vi "GUI.vi"() -> ()   [LabVIEW 2025]
uses:
  Data.ctl
  Case.ctl
  <vilib>/httpClient/ClientHandle.ctl
  User Connections/User Connections.lvclass
  Ini File/Ini File.lvclass
  D:/Repository/Semaphore-with-ESP32-C6/LabVIEW/User Connections/User Connections.lvclass
  <vilib>/JDP Science/JSONtext/Next JSON Value.vi
  <vilib>/JDP Science/JSONtext/String Subset.vi
  <vilib>/JDP Science/JSONtext/Parsing/Advance past next JSON Value (inlined COPY).vi
  <vilib>/JDP Science/JSONtext/Parsing/Advance past whitespace.vi
  <vilib>/JDP Science/JSONtext/Parsing/Advance past String.vi
  <vilib>/JDP Science/JSONtext/Parsing/Advance past Number.vi
  <vilib>/JDP Science/JSONtext/Parsing/Advance past Line Ending.vi
  <vilib>/JDP Science/JSONtext/Parsing/Parse Full Path or Item Name.vi
  <vilib>/JDP Science/JSONtext/Parsing/Advance past Array.vi
  <vilib>/JDP Science/JSONtext/Parsing/Advance past Object.vi
  <vilib>/JDP Science/JSONtext/support/Error Cluster From Code.vi
  <vilib>/JDP Science/JSONtext/Offset/Find Item Locations by Path.vi
  <vilib>/httpClient/POSTBuffer.vi
  <vilib>/httpClient/LabVIEWHTTPClient.lvlib
  <vilib>/JDP Science/JSONtext/JSONtext.lvlib
panel:
  in  "status":bool caption="0"
  out "Note":string
  out "While":bool caption="4"
  in  "IP Address":string="127.0.0.1"
  out "Red":bool caption="3"
  out "Yellow":bool caption="2"
  out "Green":bool caption="1"
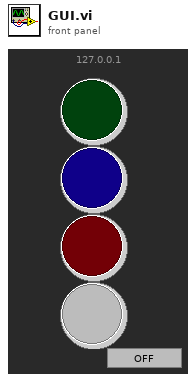
[diagram p1: front panel]
types:
  T1 = typedef "Data.ctl" = cluster{"Enum":T2, "Data":variant}
  T2 = typedef "Case.ctl" = enum16{"Initialize", "ReadFile", "LightStatus", "Parsing light", "Change light", "Close", "Change ip", "Connection"}
  T3 = typedef "LabVIEWHTTPClient.lvlib/ClientHandle.ctl" = refnum<k1>
  T4 = cluster{"IP Address":string, "timeout (10000)":i32, "client":T3, "body":string, "url":string, "File Library":refnum<class "User Connections.lvclass">}
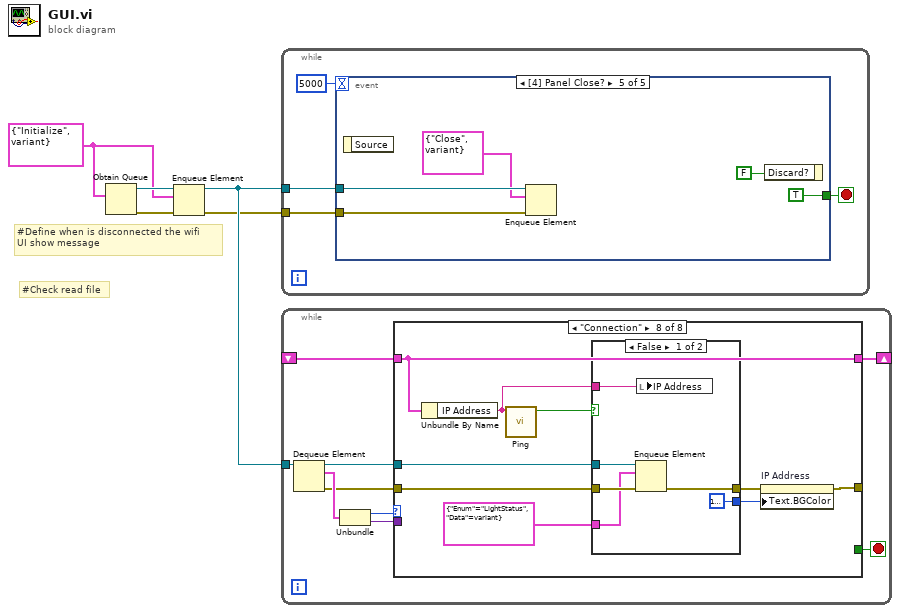
[diagram p0: block diagram]
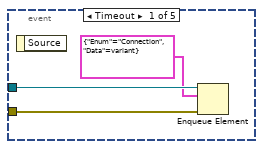
[diagram p2: hidden frame]
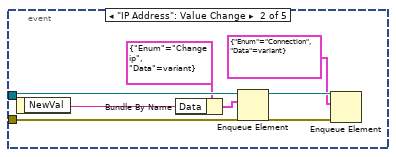
[diagram p3: hidden frame]
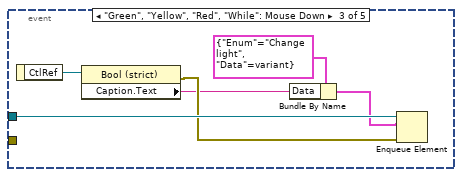
[diagram p4: hidden frame]
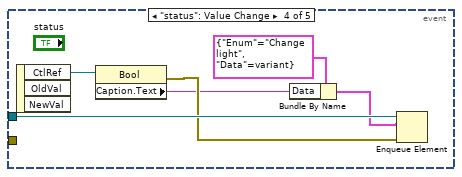
[diagram p5: hidden frame]
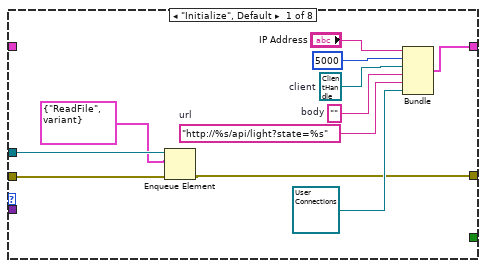
[diagram p6: hidden frame]
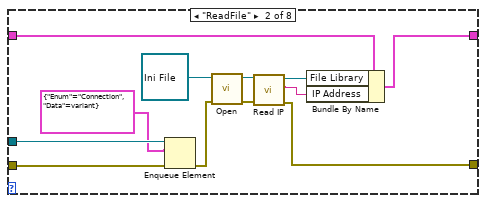
[diagram p7: hidden frame]
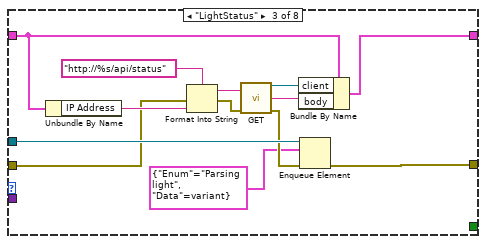
[diagram p8: hidden frame]
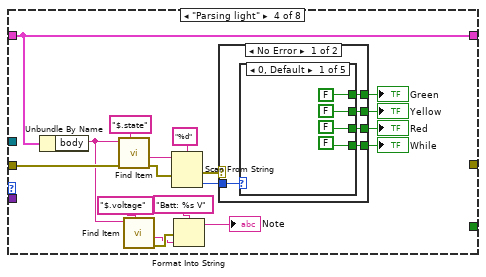
[diagram p9: hidden frame]
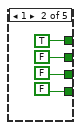
[diagram p10: hidden frame]
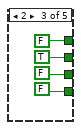
[diagram p11: hidden frame]
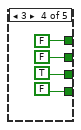
[diagram p12: hidden frame]
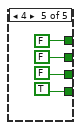
[diagram p13: hidden frame]
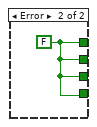
[diagram p14: hidden frame]
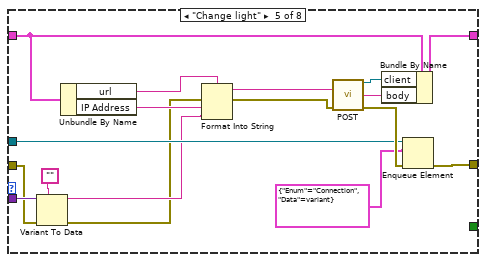
[diagram p15: hidden frame]
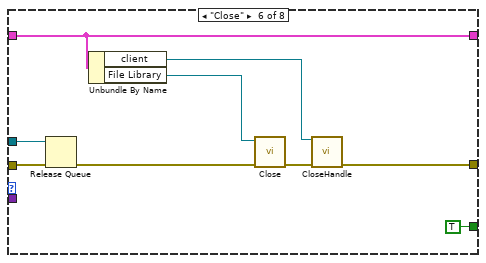
[diagram p16: hidden frame]
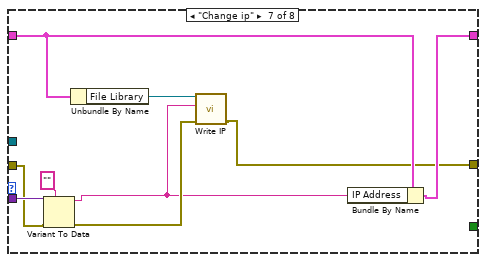
[diagram p17: hidden frame]
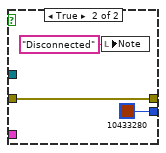
[diagram p18: hidden frame]
diagram:
  w4 = T1 {"Enum"=enum."Initialize", "Data"=variant} ("Message")
  # "#Check read file"
  # "#Define when is disconnected the wifi\nUI show message"
  n1 = Obtain Queue(element data type=w4) -> (queue out=w5:refnum<queue>, error out=w3:errorcluster)  [unwired: 4 in, 1 out]
  n2 = Enqueue Element(queue=w5, element=w4, error in (no error)=w3) -> (queue out=w2:refnum<queue>, error out=w1:errorcluster)  [unwired: 1 in, 1 out]
  n3 = while {
    tunnel: w2 -> [w8]
    tunnel: w1 -> [w7]
    stop <- w9 stop-if-true
    n4 = event shown="[4] Panel Close?" {
      selector: _ -> [_ _ _ _ _]
      dyn-events: _ -> [_ _ _ _ _]
      timeout: 5000 -> [_ _ _ _ _]
      tunnel: [_ _ _ _ TRUE ("Discard?")] -> w9
      tunnel: w8 -> [w12 w19 w26 w32 w36]
      tunnel: w7 -> [w11 w20 _ _ w35]
      event Timeout {
        n5 = event-data() -> ()  [unwired: 1 in, 1 out]
        n6 = Enqueue Element(queue=w12, element=T1 {"Enum"=enum."Connection", "Data"=variant} ("Message"), error in (no error)=w11) -> ()  [unwired: 1 in, 3 out]
      }
      event "IP Address": Value Change {
        n7 = event-data() -> ("NewVal"=w16:string)  [unwired: 1 in]
        n8 = Bundle By Name(cluster=T1 {"Enum"=enum."Change ip", "Data"=variant} ("Message"), "Data"=w16) -> (w17:T1)
        n9 = Enqueue Element(queue=w19, element=w17, error in (no error)=w20) -> (queue out=w15:refnum<queue>, error out=w14:errorcluster)  [unwired: 1 in, 1 out]
        n10 = Enqueue Element(queue=w15, element=T1 {"Enum"=enum."Connection", "Data"=variant} ("Message"), error in (no error)=w14) -> ()  [unwired: 1 in, 3 out]
      }
      event "Green", "Yellow", "Red", "While": Mouse Down {
        n11 = event-data() -> ("CtlRef"=w25:refnum<vi>)  [unwired: 1 in]
        n12 = property class="Bool (strict)"(reference=w25) -> (error out=w24:errorcluster, "Caption.Text"=w22:string)  [unwired: 1 in, 1 out]
        n13 = Bundle By Name(cluster=T1 {"Enum"=enum."Change light", "Data"=variant} ("Message"), "Data"=w22) -> (w21:T1)
        n14 = Enqueue Element(queue=w26, element=w21, error in (no error)=w24) -> ()  [unwired: 1 in, 3 out]
      }
      event "status": Value Change {
        n15 = event-data() -> ("CtlRef"=w31:refnum<vi>)  [unwired: 1 in, 2 out]
        n16 = property class="Bool"(reference=w31) -> (error out=w30:errorcluster, "Caption.Text"=w28:string)  [unwired: 1 in, 1 out]
        n17 = Bundle By Name(cluster=T1 {"Enum"=enum."Change light", "Data"=variant} ("Message"), "Data"=w28) -> (w27:T1)
        n18 = Enqueue Element(queue=w32, element=w27, error in (no error)=w30) -> ()  [unwired: 1 in, 3 out]
      }
      event Panel Close? {
        n19 = event-data() -> ()  [unwired: 1 in, 1 out]
        n20 = Enqueue Element(queue=w36, element=T1 {"Enum"=enum."Close", "Data"=variant} ("Message"), error in (no error)=w35) -> ()  [unwired: 1 in, 3 out]
        n21 = event-data("Discard?"=FALSE) -> ()  [unwired: 1 in, 1 out]
      }
    }
  }
  n22 = while {
    tunnel: w2 -> [w46]
    shift-right: [w38] -> _
    shift-left: _ -> [w39]
    stop <- w41 stop-if-true
    n23 = Dequeue Element(queue=w46) -> (queue out=w43:refnum<queue>, element=w45:T1, error out=w42:errorcluster)  [unwired: 2 in, 1 out]
    n24 = Unbundle(w45) -> ("Enum"=w44:T2, "Data"=w40:variant)
    n25 = case shown="\"Connection\"" w44 {
      tunnel: w43 -> [w56 w69 w82 _ w141 w152 _ w166]
      tunnel: w42 -> [w55 w68 w72 w99 w129 w151 w158 w165]
      tunnel: [_ _ _ _ _ TRUE _ _] -> w41
      tunnel: w40 -> [_ _ _ _ w135 _ w161 _]
      tunnel: w39 -> [_ w66 w80 w100 w143 w149 w157 w170]
      tunnel: [w57 w65 w77 w100 w138 w149 w159 w170] -> w38
      tunnel: [w47 w58 w70 _ w127 w144 w153 w167] -> _
      frame "Initialize", Default {
        w49 = "http://%s/api/light?state=%s"  # url
        w51 = ""  # body
        w52 = T3 refnum  # client
        n26 = Enqueue Element(queue=w56, element=T1 {"Enum"=enum."ReadFile", "Data"=variant} ("Message"), error in (no error)=w55) -> (error out=w47:errorcluster)  [unwired: 1 in, 2 out]
        n27 = Bundle("IP Address"="IP Address", "timeout (10000)"=5000, "client"=w52, "body"=w51, "url"=w49, "File Library"=refnum<class "User Connections.lvclass"> refnum) -> (w57:T4)  [unwired: 1 in]
      }
      frame "ReadFile" {
        n28 = Enqueue Element(queue=w69, element=T1 {"Enum"=enum."Connection", "Data"=variant} ("Message"), error in (no error)=w68) -> (error out=w59:errorcluster)  [unwired: 1 in, 2 out]
        n29 = call-dynamic "Open.vi"("error in (no error)"=w59, "Ini File in"=refnum<class "Ini File.lvclass"> refnum ("File Library.lvlib:Ini")) -> ("error out"=w64:errorcluster, "Ini File out"=w63:refnum<class "Ini File.lvclass">)  [unwired: 8 in]
        n30 = call-dynamic "Read IP.vi"("error in (no error)"=w64, "Ini File in"=w63) -> ("error out"=w58:errorcluster, "Read IP"=w60:string, "Ini File out"=w61:refnum<class "Ini File.lvclass">)  [unwired: 7 in]
        n31 = Bundle By Name(cluster=w66, "File Library"=w61, "IP Address"=w60) -> (w65:T4)
      }
      frame "LightStatus" {
        n32 = Unbundle By Name(w80) -> ("IP Address"=w79:string)
        n33 = Format Into String(format string="http://%s/api/status" ("url"), error in=w72, w79) -> (resulting string=w81:string, error out=w73:errorcluster)  [unwired: 1 in]
        n34 = call <vilib>:"GET.vi"("url"=w81, "error in (no error)"=w73) -> ("client handle out"=w76:T3, "body"=w75:string, "error out"=w78:errorcluster)  [unwired: 10 in, 1 out]
        n35 = Bundle By Name(cluster=w80, "client"=w76, "body"=w75) -> (w77:T4)
        n36 = Enqueue Element(queue=w82, element=T1 {"Enum"=enum."Parsing light", "Data"=variant} ("Message"), error in (no error)=w78) -> (error out=w70:errorcluster)  [unwired: 1 in, 2 out]
      }
      frame "Parsing light" {
        n37 = Unbundle By Name(w100) -> ("body"=w88:string)
        n38 = call <vilib>:"Find Item.vi"("$Path or Item Name"="$.state", "error in (no error)"=w99, "JSON"=w88) -> ("error out"=w96:errorcluster, "<JSON>"=w97:string)  [unwired: 5 in, 2 out]
        n39 = call <vilib>:"Find Item.vi"("$Path or Item Name"="$.voltage", "JSON"=w88) -> ("error out"=w86:errorcluster, "<JSON>"=w85:string)  [unwired: 6 in, 2 out]
        n40 = Scan From String(format string="%d" ("$Path or Item Name"), input string=w97, error in=w96) -> (error out=w95:errorcluster, output 1=w94:i32)  [unwired: 2 in, 2 out]
        n41 = Format Into String(format string="Batt: %s V", error in=w86, w85) -> (resulting string=→"Note":string)  [unwired: 1 in, 1 out]
        n42 = case shown="No Error" w95 {
          tunnel: w94 -> [w105 _]
          tunnel: [w104 w126] -> w92
          tunnel: [w103 w126] -> w91
          tunnel: [w102 w126] -> w90
          tunnel: [w101 w126] -> w89
          frame No Error {
            n43 = case shown="0, Default" w105 {
              tunnel: [FALSE TRUE FALSE FALSE FALSE] -> w104
              tunnel: [FALSE FALSE TRUE FALSE FALSE] -> w103
              tunnel: [FALSE FALSE FALSE TRUE FALSE] -> w102
              tunnel: [FALSE FALSE FALSE FALSE TRUE] -> w101
              frame 0, Default {
              }
              frame 1 {
              }
              frame 2 {
              }
              frame 3 {
              }
              frame 4 {
              }
            }
          }
          frame Error {
            w126 = FALSE
          }
        }
        "Green" <- w92
        "Yellow" <- w91
        "Red" <- w90
        "While" <- w89
      }
      frame "Change light" {
        n44 = Variant To Data(error in=w129, type="", Variant=w135) -> (data=w133:string, error out=w130:errorcluster)
        n45 = Unbundle By Name(w143) -> ("url"=w128:string, "IP Address"=w131:string)
        n46 = Format Into String(format string=w128, error in=w130, w131, w133) -> (resulting string=w139:string, error out=w132:errorcluster)  [unwired: 1 in]
        n47 = call-poly <vilib>:"POST.vi"("url"=w139, "error in (no error)"=w132) -> ("client handle out"=w136:T3, "body"=w137:string, "error out"=w142:errorcluster)  [unwired: 10 in, 1 out]
        n48 = Bundle By Name(cluster=w143, "client"=w136, "body"=w137) -> (w138:T4)
        n49 = Enqueue Element(queue=w141, element=T1 {"Enum"=enum."Connection", "Data"=variant} ("Message"), error in (no error)=w142) -> (error out=w127:errorcluster)  [unwired: 1 in, 2 out]
      }
      frame "Close" {
        n50 = Release Queue(queue=w152, error in (no error)=w151) -> (error out=w146:errorcluster)  [unwired: 1 in, 2 out]
        n51 = Unbundle By Name(w149) -> ("client"=w148:T3, "File Library"=w147:refnum<class "User Connections.lvclass">)
        n52 = call-dynamic "Close.vi"("error in (no error)"=w146, "User Connections in"=w147) -> ("error out"=w145:errorcluster)  [unwired: 9 in]
        n53 = call <vilib>:"CloseHandle.vi"("client handle"=w148, "error in (no error)"=w145) -> ("error out"=w144:errorcluster)  [unwired: 13 in]
      }
      frame "Change ip" {
        n54 = Variant To Data(error in=w158, type="" ("url"), Variant=w161) -> (data=w154:string, error out=w155:errorcluster)
        n55 = Unbundle By Name(w157) -> ("File Library"=w156:refnum<class "User Connections.lvclass">)
        n56 = call-dynamic "Write IP.vi"("error in (no error)"=w155, "IP"=w154, "User Connections in"=w156) -> ("error out"=w153:errorcluster)  [unwired: 7 in, 1 out]
        n57 = Bundle By Name(cluster=w157, "IP Address"=w154) -> (w159:T4)
      }
      frame "Connection" {
        n58 = Unbundle By Name(w170) -> ("IP Address"=w162:string)
        n59 = call "Ping.vi"("address"=w162) -> ("disconnected?"=w169:bool)  [unwired: 10 in]
        n60 = case shown="False" w169 {
          tunnel: [u32 16777216 ("Text.Text Colors:BG Color") u32 10433280 ("Text.Text Colors:BG Color")] -> w168
          tunnel: w166 -> [w175 _]
          tunnel: w165 -> [w174 w178]
          tunnel: T1 {"Enum"=enum."LightStatus", "Data"=variant} ("Message") -> [w173 _]
          tunnel: [w172 w178] -> w163
          tunnel: w162 -> [w171 _]
          frame False {
            n61 = Enqueue Element(queue=w175, element=w173, error in (no error)=w174) -> (error out=w172:errorcluster)  [unwired: 1 in, 2 out]
            n62 = local write "IP Address"(w171) -> ()
          }
          frame True {
            n63 = local write "Note"("Disconnected" ("Note")) -> ()
          }
        }
        n64 = property on="IP Address" class="Str"(error in=w163, "Text.BGColor"=w168) -> (error out=w167:errorcluster)  [unwired: 1 in, 1 out]
      }
    }
  }
